vi "Run Robot Routine.vi"(8 "error in (no error)":errorcluster, 11 "UR5 Robot in":refnum<class "UR5 Robot.lvclass">) -> (0 "error out":errorcluster, 3 "UR5 Robot out":refnum<class "UR5 Robot.lvclass">)   [LabVIEW 2018, in "UR5 Robot.lvlib" / "UR5 Robot.lvclass"]
uses:
  UR5 Robot.lvclass
  Geometric Calibration Station/Instruments/Robot.lvlibp/Robot.lvclass
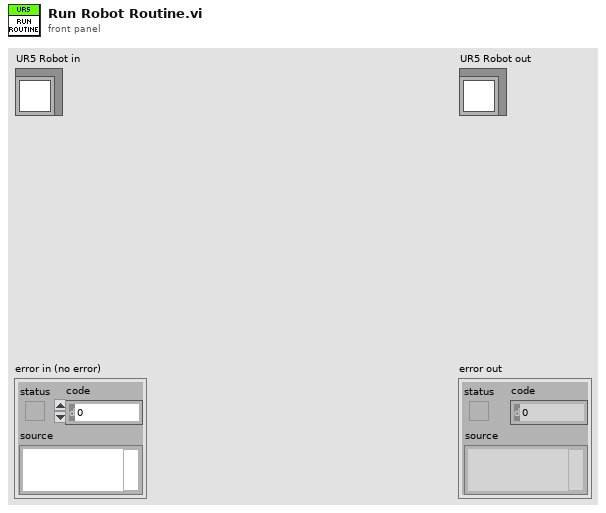
[diagram p1: front panel]
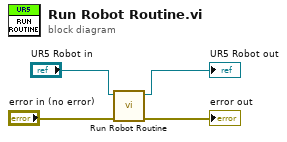
[diagram p0: block diagram]
diagram:
  n1 = call-parent "Run Robot Routine.vi"("error in (no error)"="error in (no error)", "Robot in"="UR5 Robot in") -> ("error out"=→"error out":errorcluster, "Robot out"=→"UR5 Robot out":refnum<class "UR5 Robot.lvclass">)  [unwired: 8 in]
